vi "BioIsFailed.vi"(3 "ErrorCode":dbl) -> (1 "IsFailed?":bool)   [LabVIEW 2015]
doc: "Check whether the error code belongs to fail or warning."
uses:
  Windows/System32/AdvLvDaq.dll
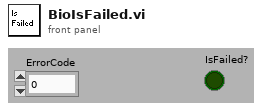
[diagram p1: front panel]
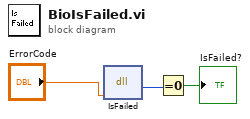
[diagram p0: block diagram]
diagram:
  n1 = dll-call lib="C:/Windows/System32/AdvLvDaq.dll" fn="IsFailed"("err"="ErrorCode") -> ("return type"=w2:i32)  [unwired: 3 in, 3 out]
  n2 = Equal To 0?(x=w2) -> (x = 0?=→"IsFailed?":bool)
